vi "monitor decimation rate t str.vi"(11 "rate":u32(ring) items=["APDM_DECIMATE_1x1", "APDM_DECIMATE_2x1", "APDM_DECIMATE_2x2", "APDM_DECIMATE_5x1", "APDM_DECIMATE_4x2", "APDM_DECIMATE_5x2", "APDM_DECIMATE_4x4", "APDM_DECIMATE_5x4", "APDM_DECIMATE_8x4", "APDM_DECIMATE_8x5", "APDM_DECIMATE_8x8"]) -> (3 "function return":string)   [LabVIEW 2019, in "apdm.lvlib"]
doc: "APDM_EXPORT const char* apdm_monitor_decimation_rate_t_str(const apdm_monitor_decimation_rate_t rate);"
uses:
  apdm.lvlib
  Lee Lab/CP FES Walking 2018/Code/Working/LabVIEW/apdm.dll
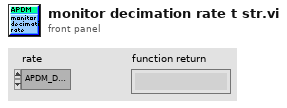
[diagram p1: front panel]
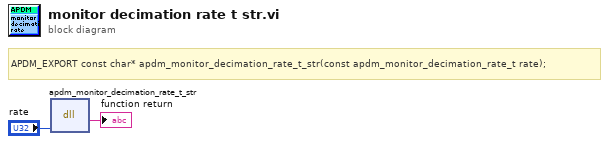
[diagram p0: block diagram]
diagram:
  # "APDM_EXPORT const char* apdm_monitor_decimation_rate_t_str(const apdm_monitor_decimation_rate_t rate);"
  n1 = dll-call lib="C:/Users/jfalesi/Dropbox/Lee Lab/CP FES Walking 2018/Code/Working/LabVIEW/apdm.*" fn="apdm_monitor_decimation_rate_t_str"("rate"="rate") -> (→"function return":string)  [unwired: 4 in, 2 out]
